vi "configuration UI.vi"() -> ()   [LabVIEW 2013, in "Logic Sequencer editor node.lvclass"]
uses:
  Logic Sequencer editor node.lvclass
  <vilib>/CEF_TreeControl/Node/NodeRef.ctl
  <vilib>/CEF_TreeControl/Node/NISE_CEF_Node.lvclass
  <vilib>/NI/AMC/Message Queue.ctl
  <vilib>/NI/AMC/Message.ctl
  <vilib>/NI/Tools/Keyed Array/KeyedArray.ctl
  <vilib>/CEF_TreeControl/Node/UserEventRef.ctl
  <vilib>/CEF_TreeControl/Controls/EventCluster.ctl
  module/configuration/processing channels.ctl
  <vilib>/NI/Tag Bus Module Framework/channel/TBM channel.lvclass
  Logic Sequencer editor node.lvclass/Logic Sequencer editor node.ctl
  <vilib>/NI/Tag Bus Module Framework/root configuration/TBM configuration.lvclass/TBM configuration.ctl
  <vilib>/NI/Tag Bus Module Framework/root configuration/create GUID.vi
  module/configuration/Logic Sequencer configuration.lvclass
  <vilib>/NI/Module Execution Interface/Engine Configuration/engine configuration.lvclass
  <vilib>/CEF_TreeControl/NISE_CEF_TreeControl.lvlib
  <vilib>/NI/Tag Bus Data Framework/Configuration Editor/Classes/Engine Parent/Engine Parent Editor Node.lvclass
  <vilib>/NI/Tag Bus Module Framework/root configuration/TBM configuration.lvclass
  <vilib>/NI/Tools/Keyed Array/Tools_KeyedArray.lvlib
  <vilib>/NI/AMC/AMC.lvlib
panel:
  in  "Tab Control":enum32{"Control Configuration"}(tab)
  in  "delete":bool
  in  "add":bool
  in  "Result Tag":u16(ring)
  in  "Parameter Tag":u16(ring)
  in  "Functions":i32(listbox)
  in  "user event":T1
  in  "main queue":T2
  in  "node ref":T3
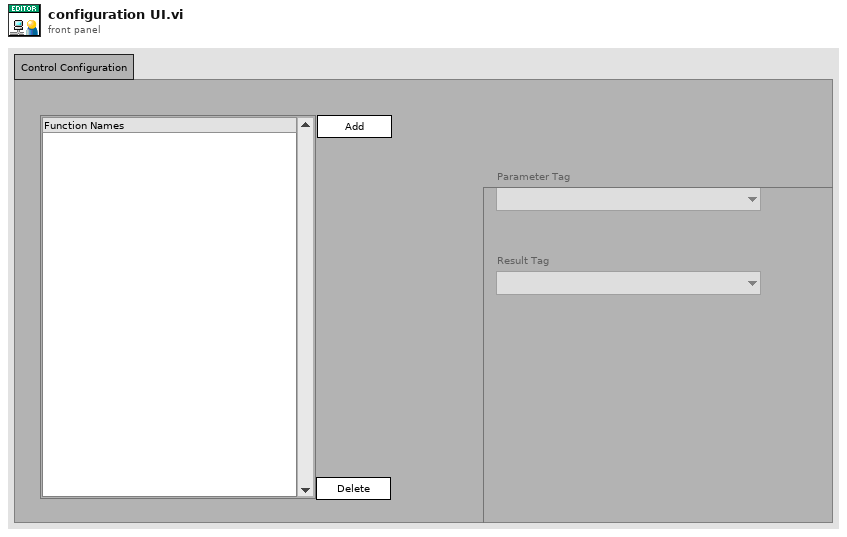
[diagram p1: front panel]
types:
  T1 = typedef "NISE_CEF_Node.lvclass/UserEventRef.ctl" = refnum<user-event>
  T2 = typedef "AMC.lvlib/Message Queue.ctl" = refnum<queue>
  T3 = typedef "NISE_CEF_Node.lvclass/NodeRef.ctl" = refnum<data-value>
  T4 = typedef "NISE_CEF_TreeControl.lvlib/EventCluster.ctl" = cluster{"command":string, "data":string}
  T5 = typedef "Logic Sequencer configuration.lvclass/processing channels.ctl" = cluster{"parameter":refnum<class "TBM channel.lvclass">, "result":refnum<class "TBM channel.lvclass">}
  T6 = enum8{"Enabled", "Disabled", "Disabled and Grayed Out"}
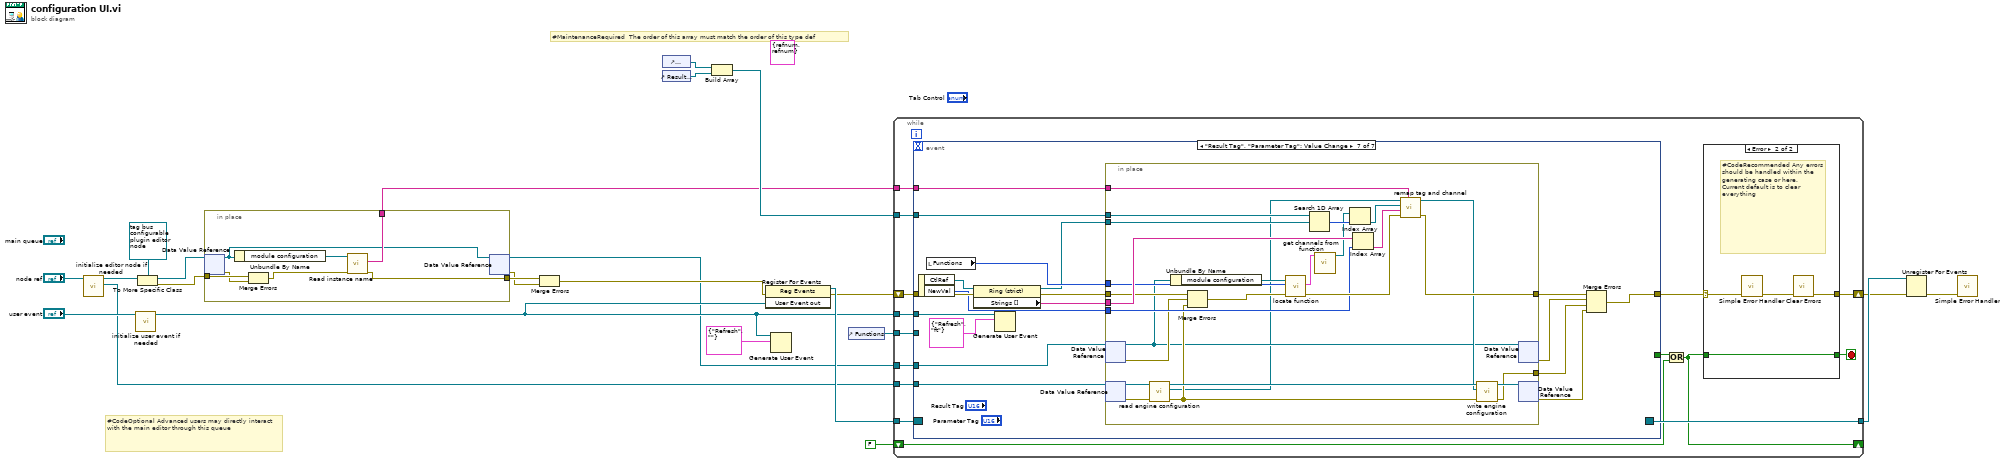
[diagram p0: block diagram]
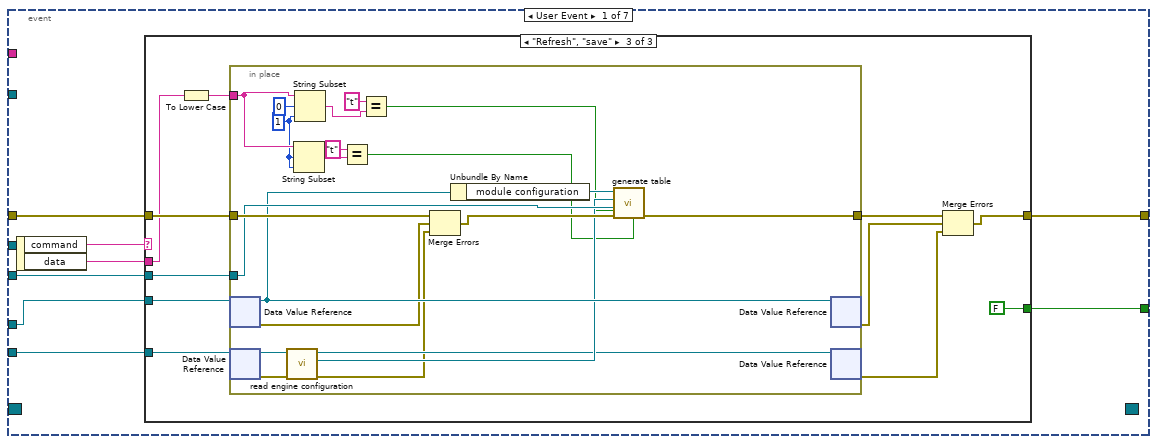
[diagram p3: hidden frame]
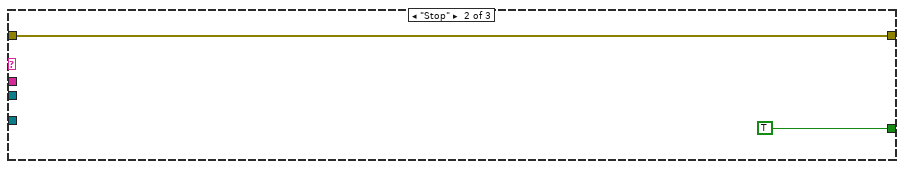
[diagram p5: hidden frame]
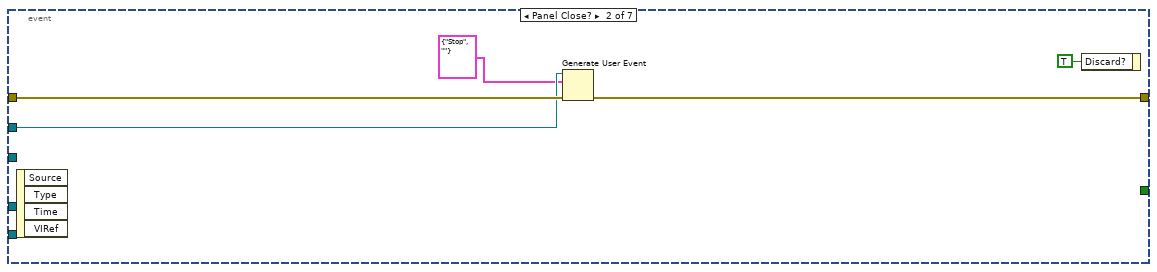
[diagram p6: hidden frame]
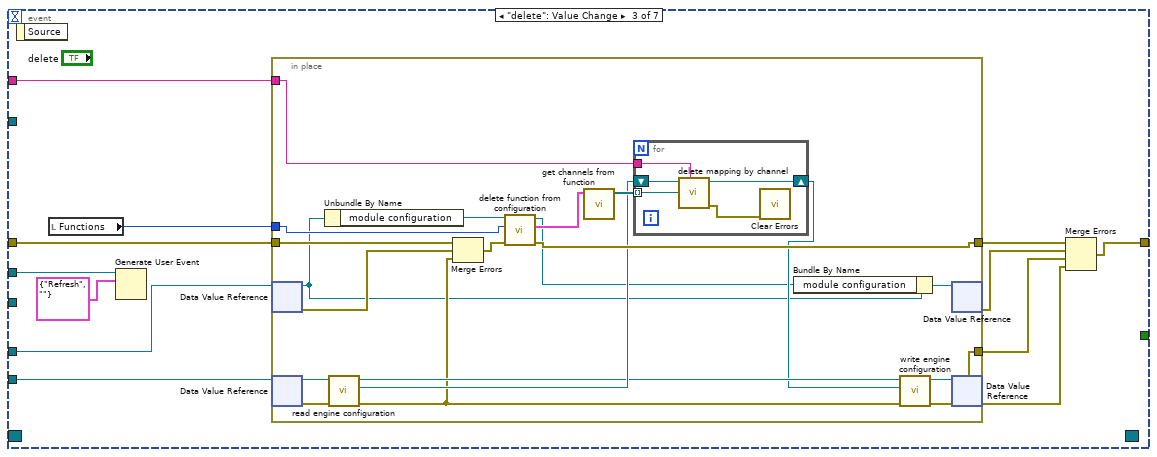
[diagram p7: hidden frame]
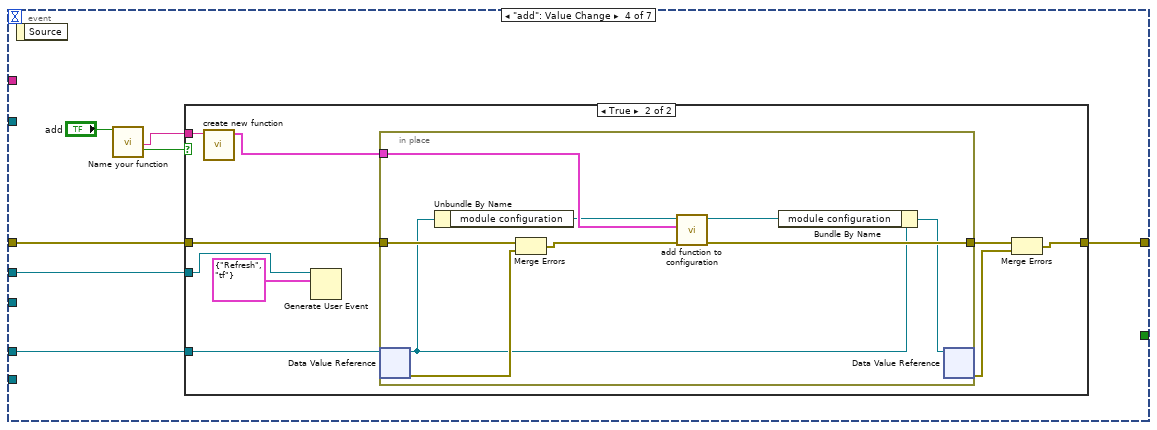
[diagram p8: hidden frame]
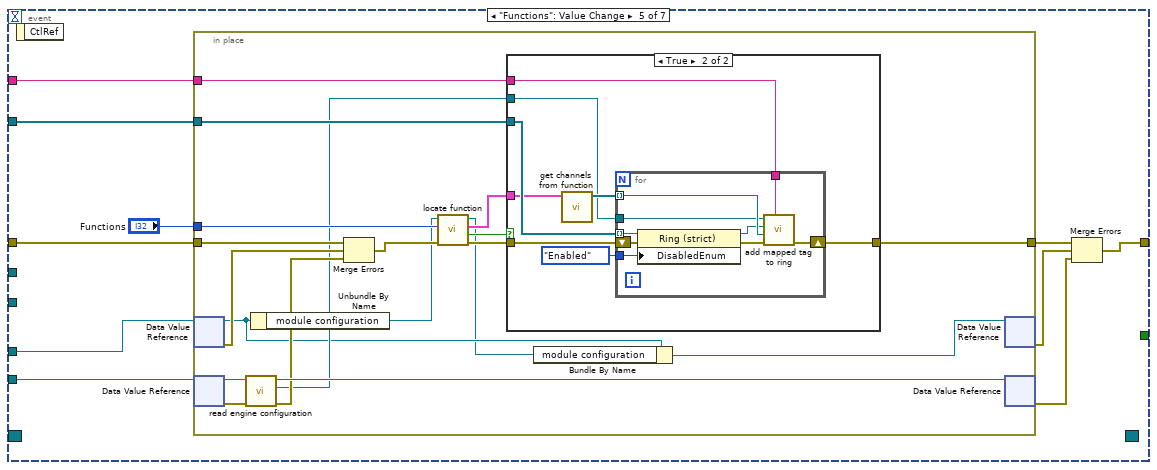
[diagram p10: hidden frame]
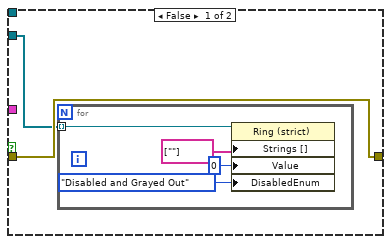
[diagram p11: hidden frame]
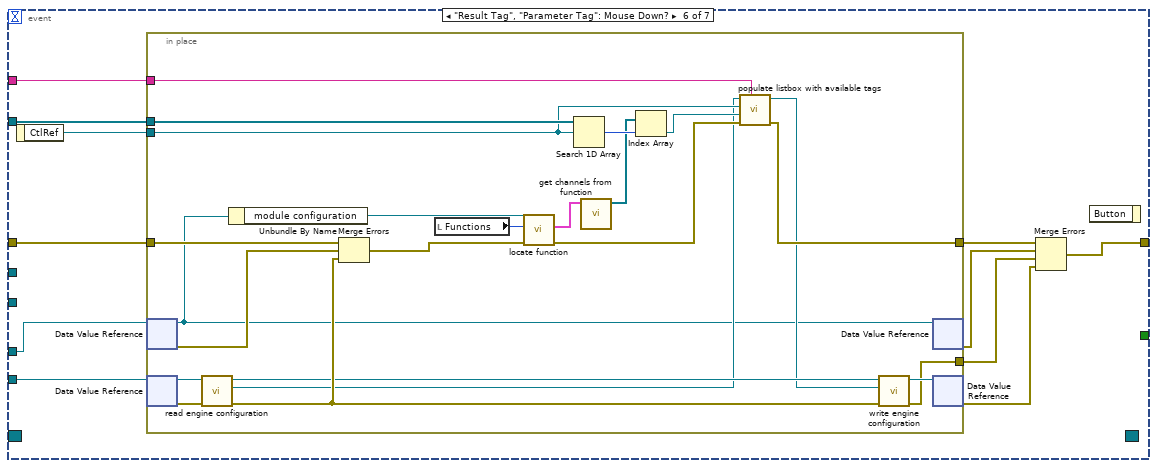
[diagram p12: hidden frame]
diagram:
  (unwired) T5 {"parameter"=refnum, "result"=refnum} ("processing function")
  # "#MaintenanceRequired  The order of this array must match the order of this type def"
  # "#CodeOptional Advanced users may directly interact with the main editor through this queue"
  n1 = call "initialize editor node if needed.vi"("editor node in"="node ref") -> ("engine"=w1:refnum<data-value>, "editor node out"=w17:T3)  [unwired: 9 in]
  n2 = call "initialize user event if needed.vi"("User Event in"="user event") -> ("User Event out"=w9:T1)  [unwired: 10 in]
  n3 = To More Specific Class(target class=refnum<data-value> refnum ("data value reference"), reference=w17) -> (specific class reference=w3:refnum<data-value>, error out=w8:errorcluster)  [unwired: 1 in]
  n4 = in-place {
    in-place-border: w8 -> [w31]
    in-place-border: [w27] -> w6
    in-place-border: [w26] -> w7
    n5 = in-place-dvr #1(w3) -> (w25:refnum<class "Logic Sequencer editor node.lvclass">, w30:errorcluster)
    n6 = Unbundle By Name(w25) -> ("module configuration"=w29:refnum<class "Logic Sequencer configuration.lvclass">)
    n7 = Merge Errors(w31, w30) -> (w28:errorcluster)
    n8 = call <vilib>:"Read instance name.vi"("error in"=w28, "configuration in"=w29) -> ("error out"=w27:errorcluster, "instance id"=w26:string)  [unwired: 7 in, 1 out]
    n9 = in-place-dvr #1(w25) -> (w2:refnum<data-value>, w5:errorcluster)
  }
  n10 = Merge Errors(w6, w5) -> (w4:errorcluster)
  n11 = control-ref of="Parameter Tag"() -> (w13:refnum<vi>)
  n12 = control-ref of="Result Tag"() -> (w12:refnum<vi>)
  n13 = Build Array(w13, w12) -> (w11:refnum<vi>[])
  n14 = register-events(error in=w4, w9) -> (reference out=w24:refnum<event-registration>, error out=w19:errorcluster)  [unwired: 1 in]
  n15 = Generate User Event(user event=w9, event data cluster=T4 {"command"="Refresh", "data"=""} ("event data")) -> ()  [unwired: 2 in, 2 out]
  n16 = control-ref of="Functions"() -> (w14:refnum<vi>)
  n17 = while {
    tunnel: w24 -> [w46]
    tunnel: [w45] -> w23
    shift-right: [w38] -> w22
    shift-left: w19 -> [w44]
    shift-right: [w40] -> _
    shift-left: FALSE -> [w39]
    tunnel: w7 -> [w37]
    tunnel: w14 -> [w36]
    tunnel: w11 -> [w35]
    tunnel: w2 -> [w34]
    tunnel: w1 -> [w33]
    tunnel: w9 -> [w32]
    stop <- w42 stop-if-true
    n18 = event shown="[6] \"Result Tag\", \"Parameter Tag\": Value Change" {
      selector: w46 -> [_ _ _ _ _ _ _]
      dyn-events: [_ _ _ _ _ _ _] -> w45
      timeout: _ -> [_ _ _ _ _ _ _]
      tunnel: [w57 _ _ _ _ _ _] -> w41
      tunnel: [w60 w99 w106 w144 w168 w221 w253] -> w43
      tunnel: w44 -> [w59 w100 w112 w143 w173 w224 w267]
      tunnel: w37 -> [_ _ w110 _ w170 w226 w264]
      tunnel: w36 -> [w54 _ _ _ _ _ _]
      tunnel: w35 -> [_ _ _ _ w169 w223 w259]
      tunnel: w34 -> [w55 _ w101 w138 w166 w219 w254]
      tunnel: w33 -> [w56 _ w105 _ w167 w220 w255]
      tunnel: w32 -> [_ w98 w107 w139 _ _ w256]
      event User Event {
        n19 = event-data() -> ("command"=w58:string, "data"=w53:string)  [unwired: 1 in]
        n20 = case shown="\"Refresh\", \"save\"" w58 {
          tunnel: [_ TRUE FALSE] -> w57
          tunnel: w55 -> [_ _ w69]
          tunnel: w56 -> [_ _ w70]
          tunnel: w59 -> [w61 w62 w73]
          tunnel: [w61 w62 w68] -> w60
          tunnel: w54 -> [_ _ w71]
          tunnel: w53 -> [_ _ w65]
          frame Default {
          }
          frame "Stop" {
          }
          frame "Refresh", "save" {
            n21 = To Lower Case(string=w65) -> (all lower case string=w64:string)
            n22 = in-place {
              in-place-border: w73 -> [w95]
              in-place-border: [w94] -> w72
              in-place-border: w71 -> [w93]
              in-place-border: w64 -> [w82]
              w81 = 1 ("length (rest)")
              n23 = in-place-dvr #2(w69) -> (w91:refnum<class "Logic Sequencer editor node.lvclass">, w84:errorcluster)
              n24 = in-place-dvr #3(w70) -> (w89:refnum<class "Engine Parent Editor Node.lvclass">, w86:errorcluster)
              n25 = call <vilib>:"read engine configuration.vi"("error in"=w86, "Engine Parent Editor Node in"=w89) -> ("error out"=w85:errorcluster, "engine configuration"=w88:refnum<class "engine configuration.lvclass">, "Engine Parent Editor Node out"=w87:refnum<class "Engine Parent Editor Node.lvclass">)  [unwired: 7 in]
              n26 = String Subset(string=w82, offset (0)=w81, length (rest)=w81) -> (substring=w80:string)
              n27 = String Subset(string=w82, offset (0)=0, length (rest)=w81) -> (substring=w77:string)
              n28 = Equal?(x="t", y=w80) -> (x = y?=w75:bool)
              n29 = Equal?(x="t", y=w77) -> (x = y?=w76:bool)
              n30 = Merge Errors(w95, w84, w85) -> (w90:errorcluster)
              n31 = Unbundle By Name(w91) -> ("module configuration"=w92:refnum<class "Logic Sequencer configuration.lvclass">)
              n32 = call "generate table.vi"("only redraw current"=w75, "select last?"=w76, "error in"=w90, "listbox"=w93, "engine configuration in"=w88, "tag bus configurable plugin module configuration in"=w92) -> ("error out"=w94:errorcluster)  [unwired: 5 in]
              n33 = in-place-dvr #2(w91) -> (w66:errorcluster)  [unwired: 1 out]
              n34 = in-place-dvr #3(w87) -> (w67:errorcluster)  [unwired: 1 out]
            }
            n35 = Merge Errors(w72, w66, w67) -> (w68:errorcluster)
          }
        }
      }
      event Panel Close? {
        n36 = event-data() -> ()  [unwired: 1 in, 4 out]
        n37 = Generate User Event(user event=w98, event data cluster=T4 {"command"="Stop", "data"=""} ("event data"), error in=w100) -> (error out=w99:errorcluster)  [unwired: 1 in, 1 out]
        n38 = event-data("Discard?"=TRUE) -> ()  [unwired: 1 in, 1 out]
      }
      event "delete": Value Change {
        n39 = event-data() -> ()  [unwired: 1 in, 1 out]
        n40 = local read "Functions"() -> (w111:i32)
        n41 = Generate User Event(user event=w107, event data cluster=T4 {"command"="Refresh", "data"=""} ("event data")) -> ()  [unwired: 2 in, 2 out]
        n42 = in-place {
          in-place-border: w112 -> [w132]
          in-place-border: w111 -> [w131]
          in-place-border: w110 -> [w128]
          in-place-border: [w127] -> w109
          in-place-border: [w122] -> w104
          n43 = in-place-dvr #4(w101) -> (w114:refnum<class "Logic Sequencer editor node.lvclass">, w117:errorcluster)
          n44 = in-place-dvr #5(w105) -> (w125:refnum<class "Engine Parent Editor Node.lvclass">, w124:errorcluster)
          n45 = Unbundle By Name(w114) -> ("module configuration"=w116:refnum<class "Logic Sequencer configuration.lvclass">)
          n46 = call <vilib>:"read engine configuration.vi"("error in"=w124, "Engine Parent Editor Node in"=w125) -> ("error out"=w118:errorcluster, "engine configuration"=w121:refnum<class "engine configuration.lvclass">, "Engine Parent Editor Node out"=w120:refnum<class "Engine Parent Editor Node.lvclass">)  [unwired: 7 in]
          n47 = Merge Errors(w132, w117, w118) -> (w126:errorcluster)
          n48 = call "delete function from configuration.vi"("error in"=w126, "index"=w131, "Logic Sequencer configuration in"=w116) -> ("error out"=w127:errorcluster, "function deleted"=w130:T5, "Logic Sequencer configuration out"=w113:refnum<class "Logic Sequencer configuration.lvclass">)  [unwired: 6 in]
          n49 = call "get channels from function.vi"("processing function"=w130) -> ("channels"=w129:refnum<class "TBM channel.lvclass">[])  [unwired: 10 in]
          n50 = for {
            shift-right: [w134] -> w119
            shift-left: w121 -> [w137]
            tunnel: w129 -> [w136] mode=indexing
            tunnel: w128 -> [w135]
            n51 = call <vilib>:"delete mapping by channel.vi"("owner ID"=w135, "channel"=w136, "engine configuration in"=w137) -> ("error out"=w133:errorcluster, "engine configuration out"=w134:refnum<class "engine configuration.lvclass">)  [unwired: 7 in]
            n52 = call <vilib>:"Clear Errors.vi"("error in (no error)"=w133) -> ()  [unwired: 6 in, 1 out]
          }
          n53 = Bundle By Name(cluster=w114, "module configuration"=w113) -> (w115:refnum<class "Logic Sequencer editor node.lvclass">)
          n54 = call <vilib>:"write engine configuration.vi"("error in"=w118, "engine configuration"=w119, "Engine Parent Editor Node in"=w120) -> ("error out"=w122:errorcluster, "Engine Parent Editor Node out"=w123:refnum<class "Engine Parent Editor Node.lvclass">)  [unwired: 7 in]
          n55 = in-place-dvr #4(w115) -> (w103:errorcluster)  [unwired: 1 out]
          n56 = in-place-dvr #5(w123) -> (w102:errorcluster)  [unwired: 1 out]
        }
        n57 = Merge Errors(w109, w103, w104, w102) -> (w106:errorcluster)
      }
      event "add": Value Change {
        n58 = event-data() -> ()  [unwired: 1 in, 1 out]
        n59 = call "Name your function"("Enable"="add") -> ("function name"=w142:string, "OK"=w141:bool)  [unwired: 16 in, 1 out]
        n60 = case shown="True" w141 {
          tunnel: [w145 w147] -> w144
          tunnel: w143 -> [w145 w154]
          tunnel: w142 -> [_ w152]
          tunnel: w139 -> [_ w149]
          tunnel: w138 -> [_ w148]
          frame False {
          }
          frame True {
            n61 = call "create new function.vi"("function name"=w152) -> ("processing function"=w151:T5)  [unwired: 10 in]
            n62 = Generate User Event(user event=w149, event data cluster=T4 {"command"="Refresh", "data"="tf"} ("event data")) -> ()  [unwired: 2 in, 2 out]
            n63 = in-place {
              in-place-border: w154 -> [w163]
              in-place-border: [w162] -> w153
              in-place-border: w151 -> [w161]
              n64 = in-place-dvr #6(w148) -> (w157:refnum<class "Logic Sequencer editor node.lvclass">, w159:errorcluster)
              n65 = Unbundle By Name(w157) -> ("module configuration"=w155:refnum<class "Logic Sequencer configuration.lvclass">)
              n66 = Merge Errors(w163, w159) -> (w160:errorcluster)
              n67 = call "add function to configuration.vi"("error in"=w160, "processing function"=w161, "Logic Sequencer configuration in"=w155) -> ("error out"=w162:errorcluster, "Logic Sequencer configuration out"=w156:refnum<class "Logic Sequencer configuration.lvclass">)  [unwired: 7 in]
              n68 = Bundle By Name(cluster=w157, "module configuration"=w156) -> (w158:refnum<class "Logic Sequencer editor node.lvclass">)
              n69 = in-place-dvr #6(w158) -> (w146:errorcluster)  [unwired: 1 out]
            }
            n70 = Merge Errors(w153, w146) -> (w147:errorcluster)
          }
        }
      }
      event "Functions": Value Change {
        n71 = event-data() -> ()  [unwired: 1 in, 1 out]
        n72 = in-place {
          in-place-border: w173 -> [w192]
          in-place-border: "Functions" -> [w189]
          in-place-border: [w187] -> w171
          in-place-border: w170 -> [w186]
          in-place-border: w169 -> [w185]
          n73 = in-place-dvr #7(w166) -> (w176:refnum<class "Logic Sequencer editor node.lvclass">, w181:errorcluster)
          n74 = in-place-dvr #8(w167) -> (w184:refnum<class "Engine Parent Editor Node.lvclass">, w183:errorcluster)
          n75 = call <vilib>:"read engine configuration.vi"("error in"=w183, "Engine Parent Editor Node in"=w184) -> ("error out"=w179:errorcluster, "engine configuration"=w178:refnum<class "engine configuration.lvclass">, "Engine Parent Editor Node out"=w180:refnum<class "Engine Parent Editor Node.lvclass">)  [unwired: 7 in]
          n76 = Unbundle By Name(w176) -> ("module configuration"=w177:refnum<class "Logic Sequencer configuration.lvclass">)
          n77 = Merge Errors(w192, w181, w179) -> (w182:errorcluster)
          n78 = call "locate function.vi"("error in"=w182, "index"=w189, "tag bus processing plugin module configuration in"=w177) -> ("error out"=w188:errorcluster, "found"=w190:bool, "processing function"=w191:T5, "tag bus processing plugin module configuration out"=w175:refnum<class "Logic Sequencer configuration.lvclass">)  [unwired: 5 in]
          n79 = case shown="True" w190 {
            tunnel: w191 -> [_ w204]
            tunnel: w188 -> [w194 w203]
            tunnel: [w194 w200] -> w187
            tunnel: w178 -> [_ w199]
            tunnel: w186 -> [_ w201]
            tunnel: w185 -> [w193 w205]
            frame False {
              n80 = for {
                tunnel: w193 -> [w195] mode=indexing
                n81 = property on="Property Node" class="Ring (strict)"(reference=w195, "Strings []"=string[] [""], "Value"=u16 0, "DisabledEnum"=T6."Disabled and Grayed Out" ("Disabled")) -> ()  [unwired: 1 in, 2 out]
              }
            }
            frame True {
              n82 = call "get channels from function.vi"("processing function"=w204) -> ("channels"=w202:refnum<class "TBM channel.lvclass">[])  [unwired: 10 in]
              n83 = for {
                tunnel: T6."Enabled" ("Disabled") -> [w215]
                tunnel: w205 -> [w214] mode=indexing
                shift-right: [w211] -> w200
                shift-left: w203 -> [w213]
                tunnel: w202 -> [w210] mode=indexing
                tunnel: w201 -> [w208]
                tunnel: w199 -> [w207]
                n84 = property on="Property Node" class="Ring (strict)"(reference=w214, error in=w213, "DisabledEnum"=w215) -> (reference out=w209:refnum<vi>, error out=w212:errorcluster)
                n85 = call "add mapped tag to ring.vi"("instance id"=w208, "error in"=w212, "channel"=w210, "ring"=w209, "engine configuration in"=w207) -> ("error out"=w211:errorcluster)  [unwired: 5 in, 1 out]
              }
            }
          }
          n86 = Bundle By Name(cluster=w176, "module configuration"=w175) -> (w174:refnum<class "Logic Sequencer editor node.lvclass">)
          n87 = in-place-dvr #7(w174) -> (w164:errorcluster)  [unwired: 1 out]
          n88 = in-place-dvr #8(w180) -> (w165:errorcluster)  [unwired: 1 out]
        }
        n89 = Merge Errors(w171, w164, w165) -> (w168:errorcluster)
      }
      event "Result Tag", "Parameter Tag": Mouse Down? {
        n90 = event-data() -> ("CtlRef"=w222:refnum<vi>)  [unwired: 1 in]
        n91 = in-place {
          in-place-border: w226 -> [w249]
          in-place-border: [w248] -> w225
          in-place-border: w224 -> [w247]
          in-place-border: w223 -> [w244]
          in-place-border: w222 -> [w243]
          in-place-border: [w236] -> w216
          n92 = in-place-dvr #9(w219) -> (w228:refnum<class "Logic Sequencer editor node.lvclass">, w229:errorcluster)
          n93 = in-place-dvr #10(w220) -> (w235:refnum<class "Engine Parent Editor Node.lvclass">, w234:errorcluster)
          n94 = call <vilib>:"read engine configuration.vi"("error in"=w234, "Engine Parent Editor Node in"=w235) -> ("error out"=w233:errorcluster, "engine configuration"=w231:refnum<class "engine configuration.lvclass">, "Engine Parent Editor Node out"=w232:refnum<class "Engine Parent Editor Node.lvclass">)  [unwired: 7 in]
          n95 = Unbundle By Name(w228) -> ("module configuration"=w227:refnum<class "Logic Sequencer configuration.lvclass">)
          n96 = Merge Errors(w247, w229, w233) -> (w238:errorcluster)
          n97 = local read "Functions"() -> (w245:i32)
          n98 = call "locate function.vi"("error in"=w238, "index"=w245, "tag bus processing plugin module configuration in"=w227) -> ("error out"=w246:errorcluster, "processing function"=w239:T5)  [unwired: 5 in, 2 out]
          n99 = Search 1D Array(1D array=w244, element=w243) -> (index of element=w242:i32)  [unwired: 1 in]
          n100 = call "get channels from function.vi"("processing function"=w239) -> ("channels"=w241:refnum<class "TBM channel.lvclass">[])  [unwired: 10 in]
          n101 = Index Array(array=w241, index=w242) -> (element=w240:refnum<class "TBM channel.lvclass">)
          n102 = call "populate listbox with available tags.vi"("instance id"=w249, "error in"=w246, "channel"=w240, "CtlRef"=w243, "engine configuration in"=w231) -> ("error out"=w248:errorcluster, "engine configuration out"=w230:refnum<class "engine configuration.lvclass">)  [unwired: 5 in]
          n103 = call <vilib>:"write engine configuration.vi"("error in"=w233, "engine configuration"=w230, "Engine Parent Editor Node in"=w232) -> ("error out"=w236:errorcluster, "Engine Parent Editor Node out"=w237:refnum<class "Engine Parent Editor Node.lvclass">)  [unwired: 7 in]
          n104 = in-place-dvr #9(w228) -> (w217:errorcluster)  [unwired: 1 out]
          n105 = in-place-dvr #10(w237) -> (w218:errorcluster)  [unwired: 1 out]
        }
        n106 = Merge Errors(w225, w217, w216, w218) -> (w221:errorcluster)
        n107 = event-data() -> ()  [unwired: 2 in, 1 out]
      }
      event "Result Tag", "Parameter Tag": Value Change {
        n108 = event-data() -> ("CtlRef"=w266:refnum<vi>, "NewVal"=w260:u16)  [unwired: 1 in]
        n109 = local read "Functions"() -> (w263:i32)
        n110 = property class="Ring (strict)"(reference=w266, error in=w267) -> (reference out=w258:refnum<vi>, error out=w262:errorcluster, "Strings []"=w265:string[])
        n111 = Generate User Event(user event=w256, event data cluster=T4 {"command"="Refresh", "data"="ft"} ("event data")) -> ()  [unwired: 2 in, 2 out]
        n112 = in-place {
          in-place-border: w265 -> [w293]
          in-place-border: w264 -> [w292]
          in-place-border: w263 -> [w291]
          in-place-border: w262 -> [w289]
          in-place-border: [w287] -> w261
          in-place-border: w260 -> [w286]
          in-place-border: w259 -> [w285]
          in-place-border: w258 -> [w284]
          in-place-border: [w272] -> w250
          n113 = in-place-dvr #11(w254) -> (w270:refnum<class "Logic Sequencer editor node.lvclass">, w271:errorcluster)
          n114 = in-place-dvr #12(w255) -> (w278:refnum<class "Engine Parent Editor Node.lvclass">, w277:errorcluster)
          n115 = call <vilib>:"read engine configuration.vi"("error in"=w277, "Engine Parent Editor Node in"=w278) -> ("error out"=w273:errorcluster, "engine configuration"=w268:refnum<class "engine configuration.lvclass">, "Engine Parent Editor Node out"=w275:refnum<class "Engine Parent Editor Node.lvclass">)  [unwired: 7 in]
          n116 = Unbundle By Name(w270) -> ("module configuration"=w269:refnum<class "Logic Sequencer configuration.lvclass">)
          n117 = Merge Errors(w289, w271, w273) -> (w279:errorcluster)
          n118 = call "locate function.vi"("error in"=w279, "index"=w291, "tag bus processing plugin module configuration in"=w269) -> ("error out"=w290:errorcluster, "processing function"=w283:T5)  [unwired: 5 in, 2 out]
          n119 = Search 1D Array(1D array=w285, element=w284) -> (index of element=w282:i32)  [unwired: 1 in]
          n120 = call "get channels from function.vi"("processing function"=w283) -> ("channels"=w281:refnum<class "TBM channel.lvclass">[])  [unwired: 10 in]
          n121 = Index Array(array=w281, index=w282) -> (element=w280:refnum<class "TBM channel.lvclass">)
          n122 = Index Array(array=w293, index=w286) -> (element=w288:string)
          n123 = call "remap tag and channel.vi"("instance id"=w292, "error in"=w290, "tag name"=w288, "channel"=w280, "engine configuration in"=w268) -> ("error out"=w287:errorcluster, "engine configuration out"=w274:refnum<class "engine configuration.lvclass">)  [unwired: 5 in]
          n124 = call <vilib>:"write engine configuration.vi"("error in"=w273, "engine configuration"=w274, "Engine Parent Editor Node in"=w275) -> ("error out"=w272:errorcluster, "Engine Parent Editor Node out"=w276:refnum<class "Engine Parent Editor Node.lvclass">)  [unwired: 7 in]
          n125 = in-place-dvr #11(w270) -> (w251:errorcluster)  [unwired: 1 out]
          n126 = in-place-dvr #12(w276) -> (w252:errorcluster)  [unwired: 1 out]
        }
        n127 = Merge Errors(w261, w251, w250, w252) -> (w253:errorcluster)
      }
    }
    n128 = Or(x=w41, y=w39) -> (x .or. y?=w40:bool)
    n129 = case shown="Error" w43 {
      selector: w43 -> [w47 w51]
      tunnel: [w48 w52] -> w42
      tunnel: w40 -> [w48 w52]
      tunnel: [w47 w49] -> w38
      frame No Error {
      }
      frame Error {
        # "#CodeRecommended Any errors should be handled within the generating case or here. Current default is to clear everything"
        n130 = call <vilib>:"Simple Error Handler.vi"("error in (no error)"=w51) -> ("error out"=w50:errorcluster)  [unwired: 4 in, 4 out]
        n131 = call <vilib>:"Clear Errors.vi"("error in (no error)"=w50) -> ("error out"=w49:errorcluster)  [unwired: 6 in]
      }
    }
  }
  n132 = Unregister For Events(event registration refnum=w23, error in=w22) -> (error out=w15:errorcluster)
  n133 = call <vilib>:"Simple Error Handler.vi"("error in (no error)"=w15) -> ()  [unwired: 4 in, 5 out]
